vi "Delete Old PPLs From Public Documents.vi"(8 "error in":errorcluster, 11 "CD name":string) -> (0 "error out":errorcluster, 3 "Public Documents CD path":path)   [LabVIEW 2020, in "Template Tool.lvlib"]
uses:
  Template Tool.lvlib
  <vilib>/Utility/sysdir.llb/System Directory Type.ctl
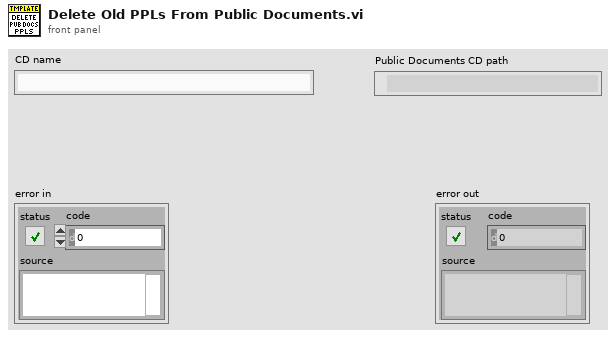
[diagram p1: front panel]
types:
  T1 = typedef "System Directory Type.ctl" = i32
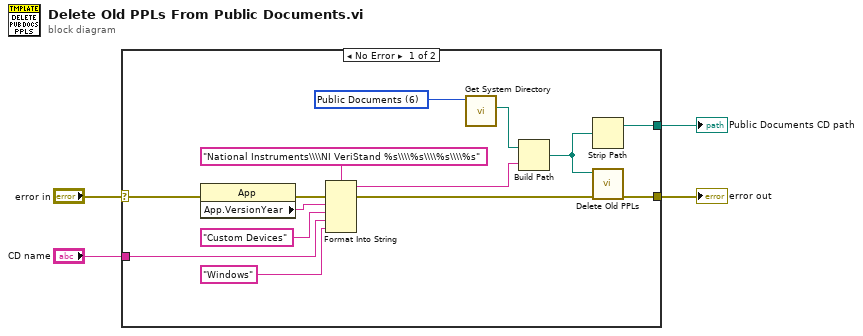
[diagram p0: block diagram]
diagram:
  n1 = case shown="No Error" "error in" {
    selector: "error in" -> [w9 w19]
    tunnel: [w18 w19] -> w4
    tunnel: "CD name" -> [w10 _]
    tunnel: [w5 _] -> w1
    frame No Error {
      w14 = T1 6 items=["User Home"=0, "User Desktop"=1, "User Documents"=2, "User Application Data"=3, "User Preferences"=4, "User Temporary"=5, "Public Documents"=6, "Public Application Data"=7, "Public Preferences"=8, "Public Cache"=13, "System Core Libraries"=9, "System Installed Libraries"=10, "Application Files"=11, "Boot Volume Root"=12] ("system directory type")
      n2 = property class="App"(error in=w9) -> (error out=w15:errorcluster, "App.VersionYear"=w16:string)  [unwired: 1 in, 1 out]
      n3 = Format Into String(format string="National Instruments\\\\NI VeriStand %s\\\\%s\\\\%s\\\\%s" ("name or relative path"), error in=w15, w16, "Custom Devices" ("CD Execution Mode"), w10, "Windows" ("CD Target")) -> (resulting string=w12:string, error out=w8:errorcluster)  [unwired: 1 in]
      n4 = call <vilib>:"Get System Directory.vi"("system directory type"=w14) -> ("system directory"=w13:path)  [unwired: 10 in]
      n5 = Build Path(base path=w13, name or relative path=w12) -> (appended path=w6:path)
      n6 = Strip Path(path=w6) -> (stripped path=w5:path)  [unwired: 1 out]
      n7 = call "Delete Old PPLs.vi"("error in"=w8, "PPLs folder path"=w6) -> ("error out"=w18:errorcluster)  [unwired: 9 in]
    }
    frame Error {
    }
  }
  "error out" <- w4
  "Public Documents CD path" <- w1
